vi "Set Op Mode.vi"(8 "error in (no error)":errorcluster, 10 "Mode":T1 items=["Operator"=0, "Engineering"=1, "Verification"=6], 11 "Acrobat Template in":refnum<class "Application.lvclass">) -> (0 "error out":errorcluster, 3 "Acrobat Template out":refnum<class "Application.lvclass">)   [LabVIEW 2017, in "Application.lvlib" / "Application.lvclass"]
uses:
  Application.lvclass
  typedefs/Op Mode -- Enum.ctl
  Application.lvclass/Application.ctl
  Properties/App Properties.lvclass
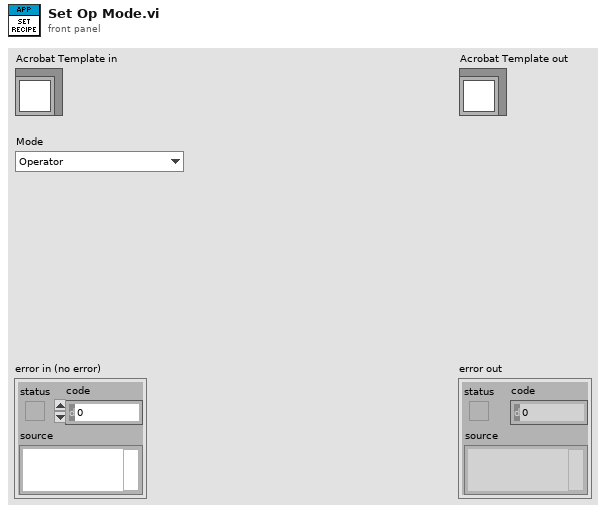
[diagram p1: front panel]
types:
  T1 = typedef "Application.lvlib/Application.lvclass/Op Mode -- Enum.ctl" = u16
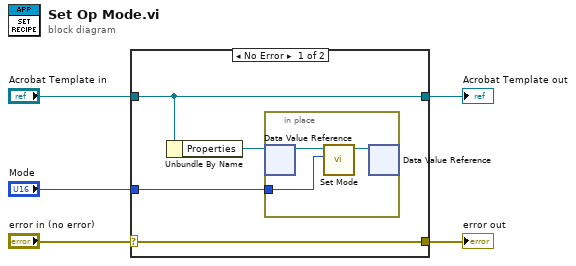
[diagram p0: block diagram]
diagram:
  n1 = case shown="No Error" "error in (no error)" {
    selector: "error in (no error)" -> [w9 w14]
    tunnel: [w9 w14] -> w4
    tunnel: [w8 w13] -> w2
    tunnel: "Acrobat Template in" -> [w8 w13]
    tunnel: "Mode" -> [w6 _]
    frame No Error {
      n2 = Unbundle By Name(w8) -> ("Properties"=w7:refnum<data-value>)
      n3 = in-place {
        in-place-border: w6 -> [w10]
        n4 = in-place-dvr #1(w7) -> (w12:refnum<class "App Properties.lvclass">)  [unwired: 1 out]
        n5 = call-dynamic "Set Mode.vi"("Mode"=w10, "App Properties in"=w12) -> ("App Properties out"=w11:refnum<class "App Properties.lvclass">)  [unwired: 8 in, 1 out]
        n6 = in-place-dvr #1(w11) -> ()  [unwired: 2 out]
      }
    }
    frame Error {
    }
  }
  "error out" <- w4
  "Acrobat Template out" <- w2
